vi "9_Compensate_Input_Delays_setInputDelay.vi"(8 "error in (no error)":errorcluster) -> (0 "error out":errorcluster)   [LabVIEW 2014]
uses:
  SwabianInstruments.TimeTagger
panel:
  in  "Clear Data":bool
  out "Counts per second":dbl[](array[numeric])
  in  "End Measurement":bool
  out "Rate":dbl[](array[numeric]) caption="Counts/s with delay adjustment"
  out "extracted delay [ps]\n (peak maximum)":i64
  out "Cross correlation":cluster{"getIndex":i64[], "getData":i32[]}(graph) caption="Cross correlation with compensated delay"
  out "Cross correlation without inputDelay adjustment":cluster{"getIndex":i64[], "getData":i32[]}(graph)
  # "STAGE 1\nThe internal test signal has a propagation delay between the \ndifferent input channels.\nThis example shows how to use setInputDelay to compensate the offset."
  # "STAGE 2\nThe internal test signal of channel 1 is now shifted from the measurement\nof STAGE 1 so that clicks of both channels arrive at the very same time."
  # "channel 1"
  # "channel 1"
  # "channel 2"
  # "channel 2"
  # "coincidences"
  # "coincidences"
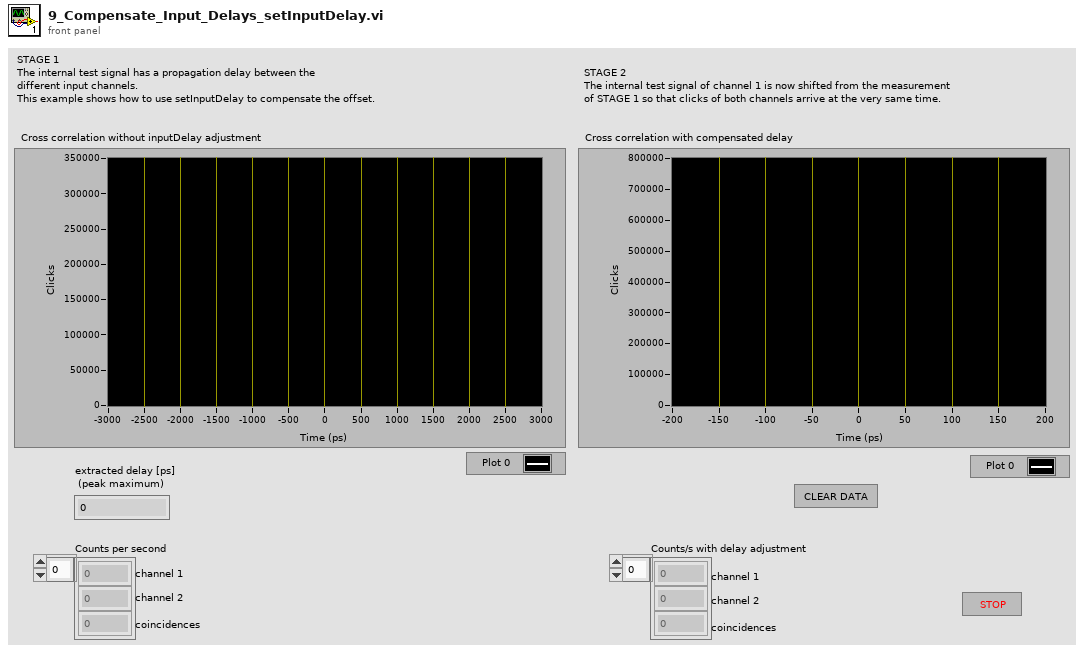
[diagram p1: front panel]
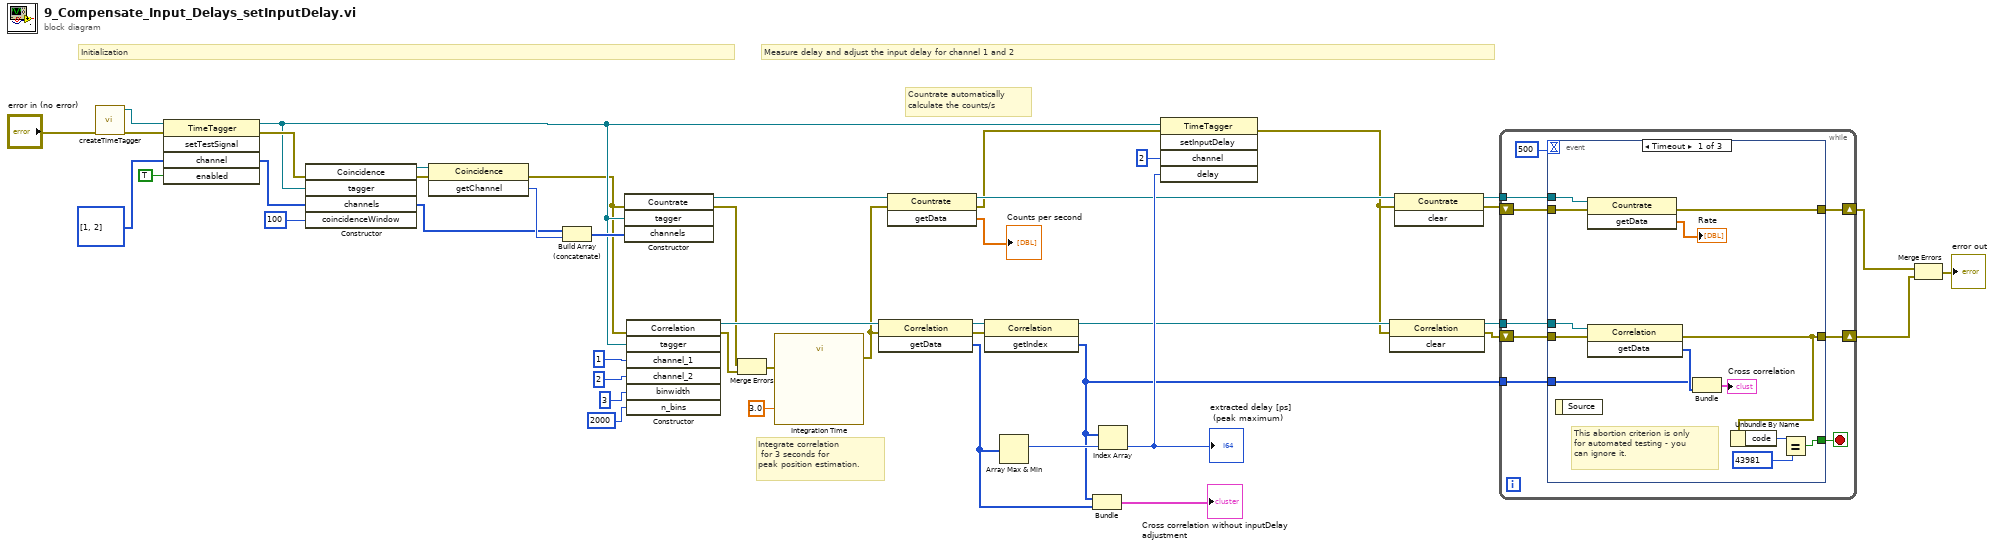
[diagram p0: block diagram]
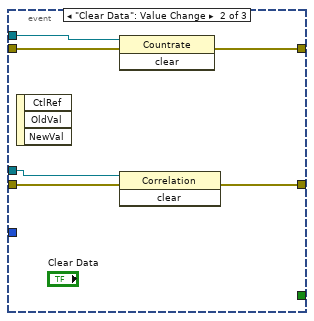
[diagram p2: hidden frame]
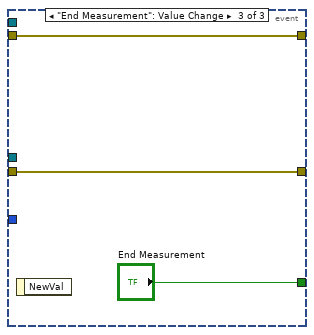
[diagram p3: hidden frame]
diagram:
  # "Integrate correlation\n for 3 seconds for\npeak position estimation."
  # "Countrate automatically \ncalculate the counts/s"
  # "Measure delay and adjust the input delay for channel 1 and 2"
  # "Initialization"
  n1 = call "createTimeTagger.vi"("error in (no error)"="error in (no error)") -> ("error out"=w19:errorcluster, "TimeTagger ref out"=w18:refnum<k24>)  [unwired: 9 in]
  n2 = invoke class="TimeTagger" method="setTestSignal"(reference=w18, error in=w19, "channel"=i32[] [1, 2], "enabled"=TRUE) -> (reference out=w7:refnum<k24>, error out=w16:errorcluster, "channel"=w13:i32[])  [unwired: 1 in, 2 out]
  n3 = constructor class="Coincidence"(error in=w16, "tagger"=w7, "channels"=w13, "coincidenceWindow"=i64 100 ("window")) -> (reference out=w22:refnum<k24>, error out=w20:errorcluster, "channels"=w14:i32[])  [unwired: 2 in, 3 out]
  n4 = invoke class="Coincidence" method="getChannel"(reference=w22, error in=w20) -> (error out=w6:errorcluster, "getChannel"=w21:i32)  [unwired: 1 in, 1 out]
  n5 = Build Array (concatenate)(w14, w21) -> (w33:i32[])
  n6 = constructor class="Countrate"(error in=w6, "tagger"=w7, "channels"=w33) -> (reference out=w26:refnum<k24>, error out=w10:errorcluster)  [unwired: 2 in, 3 out]
  n7 = constructor class="Correlation"(error in=w6, "tagger"=w7, "channel_1"=1, "channel_2"=2, "binwidth"=i64 3, "n_bins"=2000) -> (reference out=w30:refnum<k24>, error out=w9:errorcluster)  [unwired: 2 in, 6 out]
  n8 = Merge Errors(w10, w9) -> (w8:errorcluster)
  n9 = call "Integration Time"("error in (no error)"=w8, "Delay Time (s)"=3.0) -> ("error out"=w15:errorcluster)  [unwired: 9 in]
  n10 = invoke class="Correlation" method="getData"(reference=w30, error in=w15) -> (reference out=w45:refnum<k24>, error out=w27:errorcluster, "getData"=w38:i32[])  [unwired: 1 in]
  n11 = invoke class="Countrate" method="getData"(reference=w26, error in=w15) -> (reference out=w25:refnum<k24>, error out=w23:errorcluster, "getData"=→"Counts per second":dbl[])  [unwired: 1 in]
  n12 = invoke class="Correlation" method="getIndex"(reference=w45, error in=w27) -> (reference out=w31:refnum<k24>, "getIndex"=w32:i64[])  [unwired: 1 in, 1 out]
  n13 = Array Max & Min(array=w38) -> (max index (indices)=w36:i32)  [unwired: 3 out]
  n14 = Bundle("getIndex"=w32, "getData"=w38) -> (→"Cross correlation without inputDelay adjustment":cluster{"getIndex":i64[], "getData":i32[]})  [unwired: 1 in]
  n15 = Index Array(array=w32, index=w36) -> (element=w35:i64)
  "extracted delay [ps]\n (peak maximum)" <- w35
  n16 = invoke class="TimeTagger" method="setInputDelay"(reference=w7, error in=w23, "channel"=2, "delay"=w35) -> (error out=w5:errorcluster)  [unwired: 1 in, 4 out]
  n17 = invoke class="Correlation" method="clear"(reference=w31, error in=w5) -> (reference out=w29:refnum<k24>, error out=w11:errorcluster)  [unwired: 1 in, 1 out]
  n18 = invoke class="Countrate" method="clear"(reference=w25, error in=w5) -> (reference out=w28:refnum<k24>, error out=w12:errorcluster)  [unwired: 1 in, 1 out]
  n19 = while {
    tunnel: w32 -> [w55]
    tunnel: w29 -> [w54]
    tunnel: w28 -> [w53]
    shift-right: [w50] -> w3
    shift-left: w11 -> [w52]
    shift-right: [w49] -> w4
    shift-left: w12 -> [w51]
    stop <- w48 stop-if-true
    n20 = event shown="[0] Timeout" {
      selector: _ -> [_ _ _]
      dyn-events: _ -> [_ _ _]
      timeout: u32 500 ("milliseconds to wait") -> [_ _ _]
      tunnel: w55 -> [w67 _ _]
      tunnel: w54 -> [w65 w72 _]
      tunnel: w53 -> [w64 w74 _]
      tunnel: w52 -> [w62 w71 w76]
      tunnel: w51 -> [w61 w73 w75]
      tunnel: [w57 w70 w76] -> w50
      tunnel: [w60 w69 w75] -> w49
      tunnel: [w56 _ "End Measurement"] -> w48
      event Timeout {
        # "This abortion criterion is only\nfor automated testing - you\ncan ignore it."
        n21 = event-data() -> ()  [unwired: 1 in, 1 out]
        n22 = invoke class="Countrate" method="getData"(reference=w64, error in=w61) -> (error out=w60:errorcluster, "getData"=→"Rate":dbl[])  [unwired: 1 in, 1 out]
        n23 = invoke class="Correlation" method="getData"(reference=w65, error in=w62) -> (error out=w57:errorcluster, "getData"=w68:i32[])  [unwired: 1 in, 1 out]
        n24 = Bundle("getIndex"=w67, "getData"=w68) -> (→"Cross correlation":cluster{"getIndex":i64[], "getData":i32[]})  [unwired: 1 in]
        n25 = Unbundle By Name(w57) -> ("code"=w59:i32)
        n26 = Equal?(x=w59, y=43981) -> (x = y?=w56:bool)
      }
      event "Clear Data": Value Change {
        n27 = event-data() -> ()  [unwired: 1 in, 3 out]
        n28 = invoke class="Countrate" method="clear"(reference=w74, error in=w73) -> (error out=w69:errorcluster)  [unwired: 1 in, 2 out]
        n29 = invoke class="Correlation" method="clear"(reference=w72, error in=w71) -> (error out=w70:errorcluster)  [unwired: 1 in, 2 out]
      }
      event "End Measurement": Value Change {
        n30 = event-data() -> ()  [unwired: 1 in, 1 out]
      }
    }
  }
  n31 = Merge Errors(w4, w3) -> (→"error out":errorcluster)
